vi "STM_Client.vi"() -> ()   [LabVIEW 2016, in "RemoteControl.STM.lvclass"]
uses:
  RemoteControl.STM.lvclass
  <vilib>/NI/STM/SubVIs/MetaDataElement.ctl
  <vilib>/NI/STM/TCP/Read Meta Data (TCP Ref).vi
  <vilib>/NI/STM/TCP/Get Connection Reference (TCP).vi
  <vilib>/NI/STM/TCP/Read Meta Data (TCP Clst).vi
  <vilib>/NI/STM/TCP/Write Message (TCP).vi
  <vilib>/NI/STM/TCP/Read Message (TCP).vi
  <userlib>/_OpenG.lib/error/error.llb/Filter Error Codes (Array)__ogtk.vi
  <vilib>/NI/STM/NI STM.lvlib
panel:
  out "Numeric":i32
  out "value":i32
  out "messsages/s":dbl
  in  "stop":bool
  out "reponse command":string
  out "response data":string
  out "setMagnet":dbl
  out "unknown":string
  out "HELP":string[](array[string])
  in  "Command":string
  out "duration ms":u32
  in  "remote address":string
  out "meta data\n(available commands)":T1[](array[typedef])
  out "ACK":string
  in  "data to send":dbl
  out "error out":errorcluster
  # "CLIENT (API)"
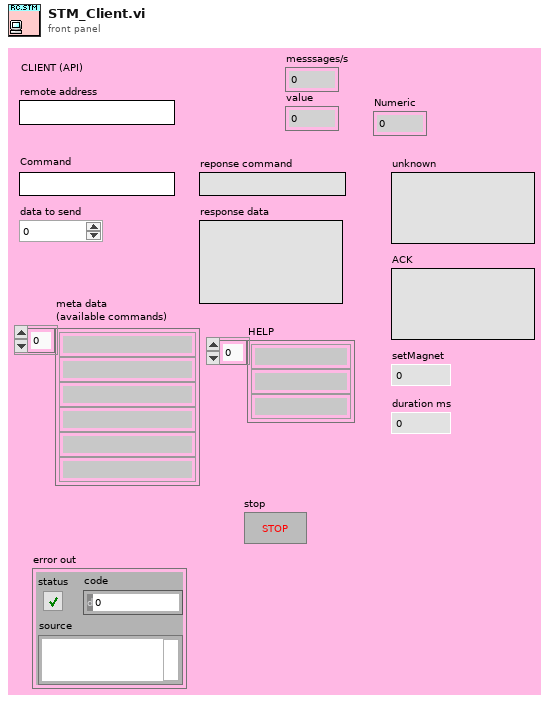
[diagram p1: front panel]
types:
  T1 = typedef "NI STM.lvlib/MetaDataElement.ctl" = string
  T2 = typedef "NI STM.lvlib/TCP Connection Info.ctl" = cluster{"connection ID":refnum<k5>, "meta data":T1[]}
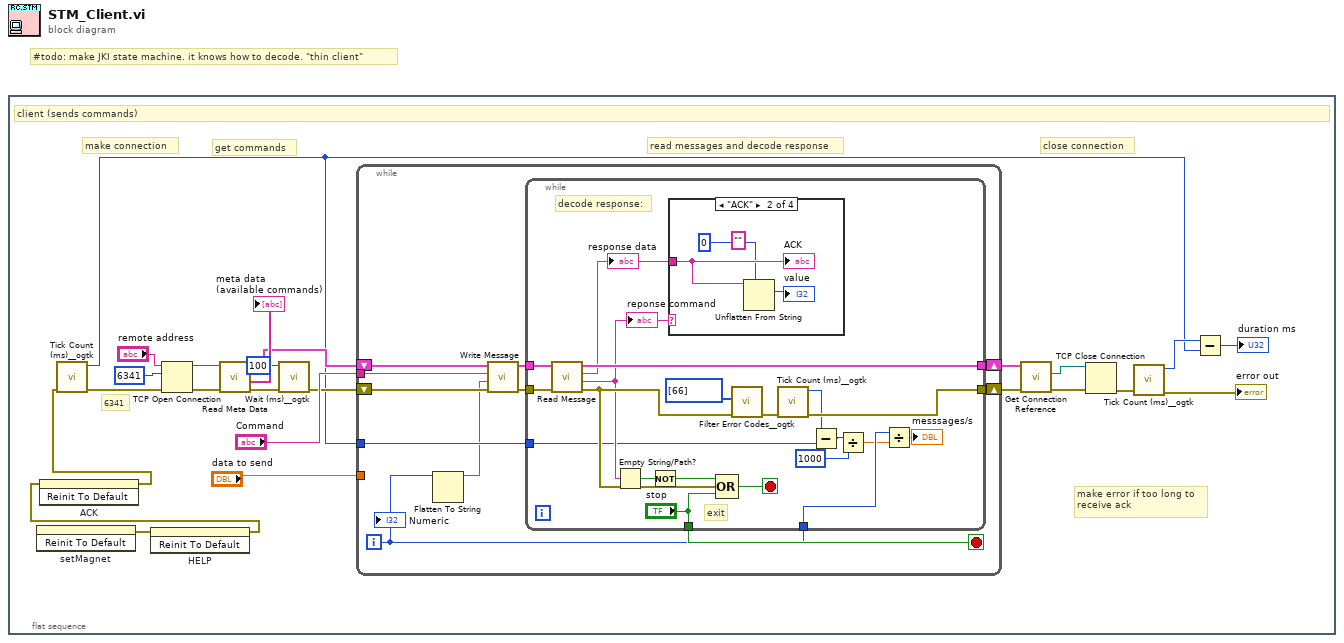
[diagram p0: block diagram]
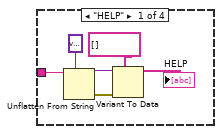
[diagram p2: hidden frame]
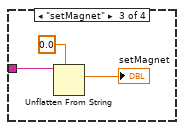
[diagram p3: hidden frame]
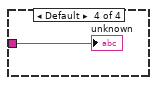
[diagram p4: hidden frame]
diagram:
  # "#todo: make JKI state machine. it knows how to decode. \"thin client\""
  n1 = flat-sequence {
    frame #0 {
      # "close connection"
      # "read messages and decode response"
      # "get commands"
      # "make connection"
      # "6341"
      # "make error if too long to\nreceive ack"
      # "client (sends commands)"
      n2 = invoke on="setMagnet" class="DigNum (strict)" method="Reinit To Default"() -> (error out=w11:errorcluster)  [unwired: 3 in, 2 out]
      n3 = invoke on="HELP" class="Arr (strict)" method="Reinit To Default"(error in=w11) -> (error out=w10:errorcluster)  [unwired: 2 in, 2 out]
      n4 = invoke on="ACK" class="Str" method="Reinit To Default"(error in=w10) -> (error out=w12:errorcluster)  [unwired: 2 in, 2 out]
      n5 = call <userlib>:"Tick Count (ms)__ogtk.vi"("error in (no error)"=w12) -> ("error out"=w19:errorcluster, "millisecond timer value"=w2:u32)  [unwired: 9 in]
      n6 = TCP Open Connection(address="remote address", remote port or service name=u16 6341, error in (no error)=w19) -> (connection ID=w23:refnum<k5>, error out=w24:errorcluster)  [unwired: 2 in]
      n7 = call-poly <vilib>:"Read Meta Data.vi"("error in"=w24, "connection ID"=w23) -> ("error out"=w6:errorcluster, "meta data"=→"meta data\n(available commands)":T1[], "connection info out"=w4:T2)  [unwired: 7 in]
      n8 = call <userlib>:"Wait (ms)__ogtk.vi"("error in (no error)"=w6, "milliseconds to wait"=u32 100) -> ("error out"=w5:errorcluster)  [unwired: 8 in, 1 out]
      n9 = while {
        tunnel: "Command" -> [w31]
        shift-right: [w33] -> w18
        shift-left: w5 -> [w30]
        shift-right: [w32] -> w17
        shift-left: w4 -> [w29]
        tunnel: w2 -> [w27]
        tunnel: "data to send" -> [_]
        i -> [w25]
        stop <- w28 stop-if-true
        n10 = Flatten To String(anything=w25) -> (data string=w26:string)  [unwired: 3 in, 2 out]
        n11 = call-poly <vilib>:"Write Message.vi"("error in"=w30, "data"=w26, "name"=w31, "connection info in"=w29) -> ("error out"=w35:errorcluster, "connection info out"=w34:T2)  [unwired: 6 in]
        n12 = while {
          tunnel: w35 -> [w55]
          tunnel: w34 -> [w54]
          tunnel: [w43] -> w33
          tunnel: [w53] -> w32
          tunnel: ["stop"] -> w28
          tunnel: w27 -> [w41]
          tunnel: w25 -> [w38]
          stop <- w52 stop-if-true
          # "decode response:"
          # "exit"
          n13 = call-poly <vilib>:"Read Message.vi"("error in"=w55, "connection info in"=w54) -> ("error out"=w51:errorcluster, "name"=w48:T1, "data string"=w49:string, "connection info out"=w53:T2)  [unwired: 2 in, 4 out]
          "response data" <- w49
          "reponse command" <- w48
          n14 = Empty String/Path?(string/path=w48) -> (empty?=w47:bool)
          n15 = Not(x=w47) -> (.not. x?=w46:bool)
          n16 = case shown="\"ACK\"" w48 {
            tunnel: w49 -> [w61 w64 w67 w68]
            frame "HELP" {
              n17 = Unflatten From String(type=variant, binary string=w61) -> (value=w58:variant, error out=w59:errorcluster)  [unwired: 3 in, 1 out]
              n18 = Variant To Data(error in=w59, type=string[] [] ("HELP"), Variant=w58) -> (data=→"HELP":string[])  [unwired: 1 out]
            }
            frame "ACK" {
              (unwired) ""
              n19 = Unflatten From String(type=0, binary string=w64) -> (value=→"value":i32)  [unwired: 3 in, 2 out]
              "ACK" <- w64
            }
            frame "setMagnet" {
              n20 = Unflatten From String(type=0.0, binary string=w67) -> (value=→"setMagnet":dbl)  [unwired: 3 in, 2 out]
            }
            frame Default {
              "unknown" <- w68
            }
          }
          n21 = Compound Arithmetic op=OR(w46, w51, "stop") -> (w52:bool)
          n22 = call-poly <userlib>:"Filter Error Codes__ogtk.vi"("Error In"=w51, "Error Codes to Filter"=i32[] [66]) -> ("Error Out"=w44:errorcluster)  [unwired: 7 in, 2 out]
          n23 = call <userlib>:"Tick Count (ms)__ogtk.vi"("error in (no error)"=w44) -> ("error out"=w43:errorcluster, "millisecond timer value"=w42:u32)  [unwired: 9 in]
          n24 = Subtract(x=w42, y=w41) -> (x-y=w40:u32)
          n25 = Divide(x=w40, y=u32 1000) -> (x/y=w37:dbl)
          n26 = Divide(x=w38, y=w37) -> (x/y=→"messsages/s":dbl)
        }
        "Numeric" <- w25
      }
      n27 = call-poly <vilib>:"Get Connection Reference.vi"("error in"=w18, "connection info in"=w17) -> ("error out"=w21:errorcluster, "connection ID out"=w20:refnum<k5>)  [unwired: 7 in, 1 out]
      n28 = TCP Close Connection(connection ID=w20, error in (no error)=w21) -> (error out=w16:errorcluster)  [unwired: 1 in, 1 out]
      n29 = call <userlib>:"Tick Count (ms)__ogtk.vi"("error in (no error)"=w16) -> ("error out"=→"error out":errorcluster, "millisecond timer value"=w13:u32)  [unwired: 9 in]
      n30 = Subtract(x=w13, y=w2) -> (x-y=→"duration ms":u32)
    }
  }
